vi "AddElevator.vi"(10 "Elevator Up":bool, 11 "Refnum in":T1) -> (3 "Refnum out":T1)   [LabVIEW 2019]
uses:
  <vilib>/vision/Image Controls.llb/IMAQ Image.ctl
  <vilib>/vision/NI_Vision_Development_Module.lvlib
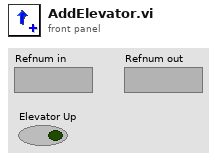
[diagram p1: front panel]
types:
  T1 = typedef "IMAQ Image.ctl" = refnum<image>
  T2 = typedef "Image Type" = u32
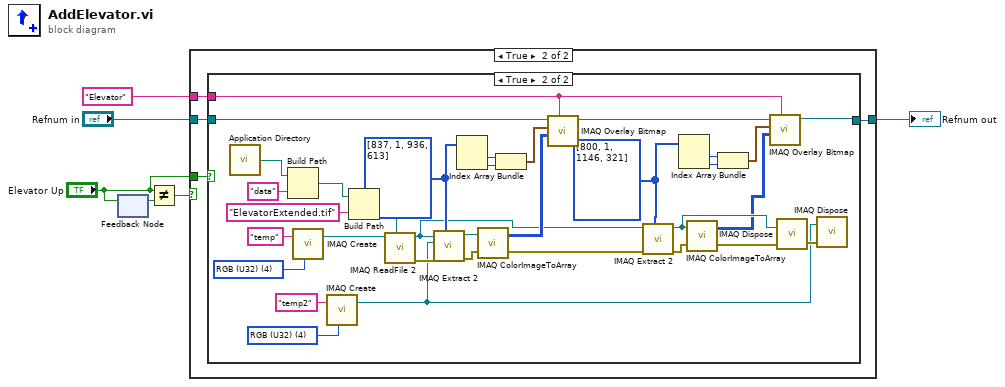
[diagram p0: block diagram]
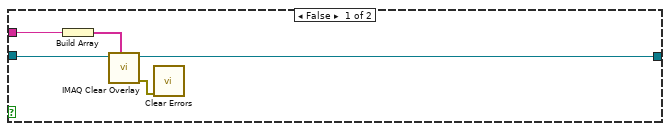
[diagram p3: hidden frame]
diagram:
  n1 = feedback-in #1("Elevator Up") -> ()
  n2 = feedback #1() -> (w5:bool)  [unwired: 1 in]
  n3 = Not Equal?(x="Elevator Up", y=w5) -> (x != y?=w6:bool)
  n4 = case shown="True" w6 {
    tunnel: [w7 w9] -> w4
    tunnel: "Refnum in" -> [w7 w10]
    tunnel: "Elevator Up" -> [_ w11]
    tunnel: "Elevator" -> [_ w8]
    frame False {
    }
    frame True {
      n5 = case shown="True" w11 {
        tunnel: w10 -> [w16 w50]
        tunnel: [w15 w20] -> w9
        tunnel: w8 -> [w14 w19]
        frame False {
          n6 = Build Array(w14) -> (w13:string[])
          n7 = call "IMAQ Clear Overlay"("Groups"=w13, "Image"=w16) -> ("error out"=w12:errorcluster, "Image Out"=w15:T1)  [unwired: 8 in]
          n8 = call <vilib>:"Clear Errors.vi"("error in (no error)"=w12) -> ()  [unwired: 5 in, 2 out]
        }
        frame True {
          w17 = i32[] [800, 1, 1146, 321] ("Optional Rectangle")
          w32 = T2 4 items=["Grayscale (U8)", "Grayscale (I16)", "Grayscale (SGL)", "Complex (CSG)", "RGB (U32)", "HSL (U32)", "RGB (U64)", "Grayscale (U16)"] ("Image Type")
          w38 = i32[] [837, 1, 936, 613] ("Optional Rectangle")
          w43 = T2 4 items=["Grayscale (U8)", "Grayscale (I16)", "Grayscale (SGL)", "Complex (CSG)", "RGB (U32)", "HSL (U32)", "RGB (U64)", "Grayscale (U16)"] ("Image Type")
          n9 = call <vilib>:"Application Directory.vi"() -> ("Application Directory"=w48:path)
          n10 = Build Path(base path=w48, name or relative path="data") -> (appended path=w49:path)
          n11 = call "IMAQ Create"("Image Name"="temp", "Image Type"=w43) -> ("New Image"=w42:T1)  [unwired: 3 in, 1 out]
          n12 = call "IMAQ Create"("Image Name"="temp2", "Image Type"=w32) -> ("New Image"=w25:T1)  [unwired: 3 in, 1 out]
          n13 = Build Path(base path=w49, name or relative path="ElevatorExtended.tif") -> (appended path=w45:path)
          n14 = call "IMAQ ReadFile 2"("File Path"=w45, "Image"=w42) -> ("error out"=w41:errorcluster, "Image Out"=w28:T1)  [unwired: 5 in, 3 out]
          n15 = call "IMAQ Extract 2"("Optional Rectangle"=w38, "error in (no error)"=w41, "Image Dst"=w25, "Image Src"=w28) -> ("error out"=w40:errorcluster, "Image Dst Out"=w34:T1)  [unwired: 6 in]
          n16 = Index Array(array=w38) -> (element #1=w36:i32, element #2=w37:i32)  [unwired: 2 in]
          n17 = call "IMAQ ColorImageToArray"("Image"=w34, "error in (no error)"=w40) -> ("Image Pixels (U32)"=w39:u32[][], "error out"=w27:errorcluster)  [unwired: 2 in, 1 out]
          n18 = Bundle(w36, w37) -> (w35:cluster{i32, i32})  [unwired: 1 in]
          n19 = call "IMAQ Overlay Bitmap"("Group"=w19, "Bitmap"=w39, "Top Left Point"=w35, "Image"=w50) -> ("Image Out"=w21:T1)  [unwired: 6 in, 1 out]
          n20 = call "IMAQ Extract 2"("Optional Rectangle"=w17, "error in (no error)"=w27, "Image Src"=w28) -> ("error out"=w29:errorcluster, "Image Dst Out"=w31:T1)  [unwired: 7 in]
          n21 = Index Array(array=w17) -> (element #1=w23:i32, element #2=w22:i32)  [unwired: 2 in]
          n22 = call "IMAQ ColorImageToArray"("Image"=w31, "error in (no error)"=w29) -> ("Image Pixels (U32)"=w18:u32[][], "error out"=w30:errorcluster)  [unwired: 2 in, 1 out]
          n23 = Bundle(w23, w22) -> (w24:cluster{i32, i32})  [unwired: 1 in]
          n24 = call "IMAQ Overlay Bitmap"("Group"=w19, "Bitmap"=w18, "Top Left Point"=w24, "Image"=w21) -> ("Image Out"=w20:T1)  [unwired: 6 in, 1 out]
          n25 = call "IMAQ Dispose"("Image"=w31, "error in (no error)"=w30) -> ("error out"=w26:errorcluster)  [unwired: 4 in]
          n26 = call "IMAQ Dispose"("Image"=w25, "error in (no error)"=w26) -> ()  [unwired: 4 in, 1 out]
        }
      }
    }
  }
  "Refnum out" <- w4
